vi "Vision Processing.vi"(4 "error in (no error)":errorcluster, 7 "Image Size":T4=enum."320x240") -> ()   [LabVIEW 2014]
doc: "This VI runs in parallel to other tasks. It gets images from the camera, processes them for color or shape and use that information to affect robot behavior."
uses:
  <vilib>/Rock Robotics/WPI/Camera/WPI_CameraImageSize.ctl
  <vilib>/Rock Robotics/WPI/Camera/WPI_CameraSettings Read MJPG.ctl
  Global Variables.vi
  Robot Global Data.vi
  <vilib>/Rock Robotics/WPI/Camera/WPI_CameraWhite Balance Values.ctl
  <vilib>/Rock Robotics/WPI/Camera/WPI_CameraExposure Values.ctl
  <vilib>/Rock Robotics/WPI/Camera/WPI_CameraFrameRate.ctl
  <vilib>/vision/NI_Vision_Development_Module.lvlib
  <vilib>/vision/Image Controls.llb/IMAQ Image.ctl
panel:
  in  "Instructions:":string="Use the tab immediately below to choose the image source. Update the camera settings or the image directory so that you have images or video to test with.\n\nCalibration:\nYou can update Color Component ranges directly, or by clicking and drawing a line across the upper third of a ball within the image -- example shown below-right.\n\nUse Debugging tab to view intermediate results. Adjust Std Dev multipliers and line to achieve the desired HSV upper and lower threshold limits.\n\nArea Size LImit is used to ignore objects too small or balls too far away to care about.\n\nTargets identifies how many of the top scores to return.\n\nThe Details tab contains center, radius, and score details of each object."
  in  "Tabbed Info":enum32{"Debugging", "Details"}(tab)
  in  "Annotations":enum16{"None", "Good", "All"}(ring)=enum."Good"
  out "Initial Mask":T1(plugin-control)
  out "Fitted Mask":T1(plugin-control)
  out "Ranked Objects":T2(array[cluster]) {"Score" format="%#.1g"}
  out "Image":T1(plugin-control)
  in  "Image Source":enum32{"Files", "Camera"}(tab)
  in  "List of image files":i32(listbox)
  in  "Image Directory":path=path "2014 Vision Target"
  in  "Camera Settings":T3={"fps"=15, "compression"=5, "Image Size"=enum."320x240"}
  in  "Camera IP":string="10.04.19.11"
  in  "Camera Address":string="192.168.0.90"
  out "Error":bool
  in  "Area Size Limit %":dbl=0.4 format="%#_13g"
  in  "Score Cutoff":dbl(slide)=70.58823529411765 scale=0.0..100.0
  out "loop time ms":u32
  in  "Targets":i32=3
  in  "Color Components":T5={"Hue"={45.217481128107224, 100.83905198430494}, "Sat"={154.78571428571428, 255.0}, "Val"={197.32142857142856, 255.0}} {"Val" scale=0.0..255.0; "Sat" scale=0.0..255.0; "Hue" scale=0.0..255.0 scale format="%#_3g"}
  in  "Std Devs":cluster{"Hue":dbl, "Sat":dbl, "Val":dbl}={"Hue"=4.0, "Sat"=6.0, "Val"=4.0}
  in  "Image Size 2":T4=enum."320x240"
  out "Blue 3":cluster{"Lower value":i32, "Upper value":i32}={"Lower value"=0, "Upper value"=255}
  out "Red":cluster{"Lower value":i32, "Upper value":i32}={"Lower value"=0, "Upper value"=255}
  out "Green 3":cluster{"Lower value":i32, "Upper value":i32}={"Lower value"=0, "Upper value"=255}
  in  "Threshold Distance":cluster{"Lower value":i32, "Upper value":i32}={"Lower value"=0, "Upper value"=255} {"Upper value" scale=0.0..255.0; "Lower value" scale=0.0..255.0}
  in  "Red Control":cluster{"Lower value":i32, "Upper value":i32}={"Lower value"=0, "Upper value"=255} {"Upper value" scale=0.0..255.0; "Lower value" scale=0.0..255.0}
  in  "Green Control":cluster{"Lower value":i32, "Upper value":i32}={"Lower value"=0, "Upper value"=255} {"Upper value" scale=0.0..255.0; "Lower value" scale=0.0..255.0}
  in  "Blue Control":cluster{"Lower value":i32, "Upper value":i32}={"Lower value"=0, "Upper value"=255} {"Upper value" scale=0.0..255.0; "Lower value" scale=0.0..255.0}
  in  "Images":T6(tab)=enum."5. Morphological Reconstruction"
  out "Source Image":T1(plugin-control)
  out "Threshold Image":T1(plugin-control)
  out "Distance Image":T1(plugin-control)
  out "Threshold Distance 2":T1(plugin-control)
  out "Reconstructed Image":T1(plugin-control)
  out "Red 2":cluster{"Lower value":i32, "Upper value":i32}={"Lower value"=0, "Upper value"=255}
  out "Blue 2":cluster{"Lower value":i32, "Upper value":i32}={"Lower value"=0, "Upper value"=255}
  out "Green 2":cluster{"Lower value":i32, "Upper value":i32}={"Lower value"=0, "Upper value"=255}
  in  "Blue":cluster{"Lower value":i32, "Upper value":i32}={"Lower value"=0, "Upper value"=255} {"Upper value" scale=0.0..255.0; "Lower value" scale=0.0..255.0}
  in  "Green":cluster{"Lower value":i32, "Upper value":i32}={"Lower value"=0, "Upper value"=255} {"Upper value" scale=0.0..255.0; "Lower value" scale=0.0..255.0}
  in  "Red or Hue Range":cluster{"Lower value":i32, "Upper value":i32}={"Lower value"=0, "Upper value"=255} {"Upper value" scale=0.0..255.0; "Lower value" scale=0.0..255.0}
  in  "Replace Value":sgl=1.0 format="%.2f"
  out "Image Dst Out":T1(plugin-control)
  out "Image Out":T1(plugin-control)
  # "Ranking Colors:\n1. green\n2. cyan\n3. magenta\n4. orange"
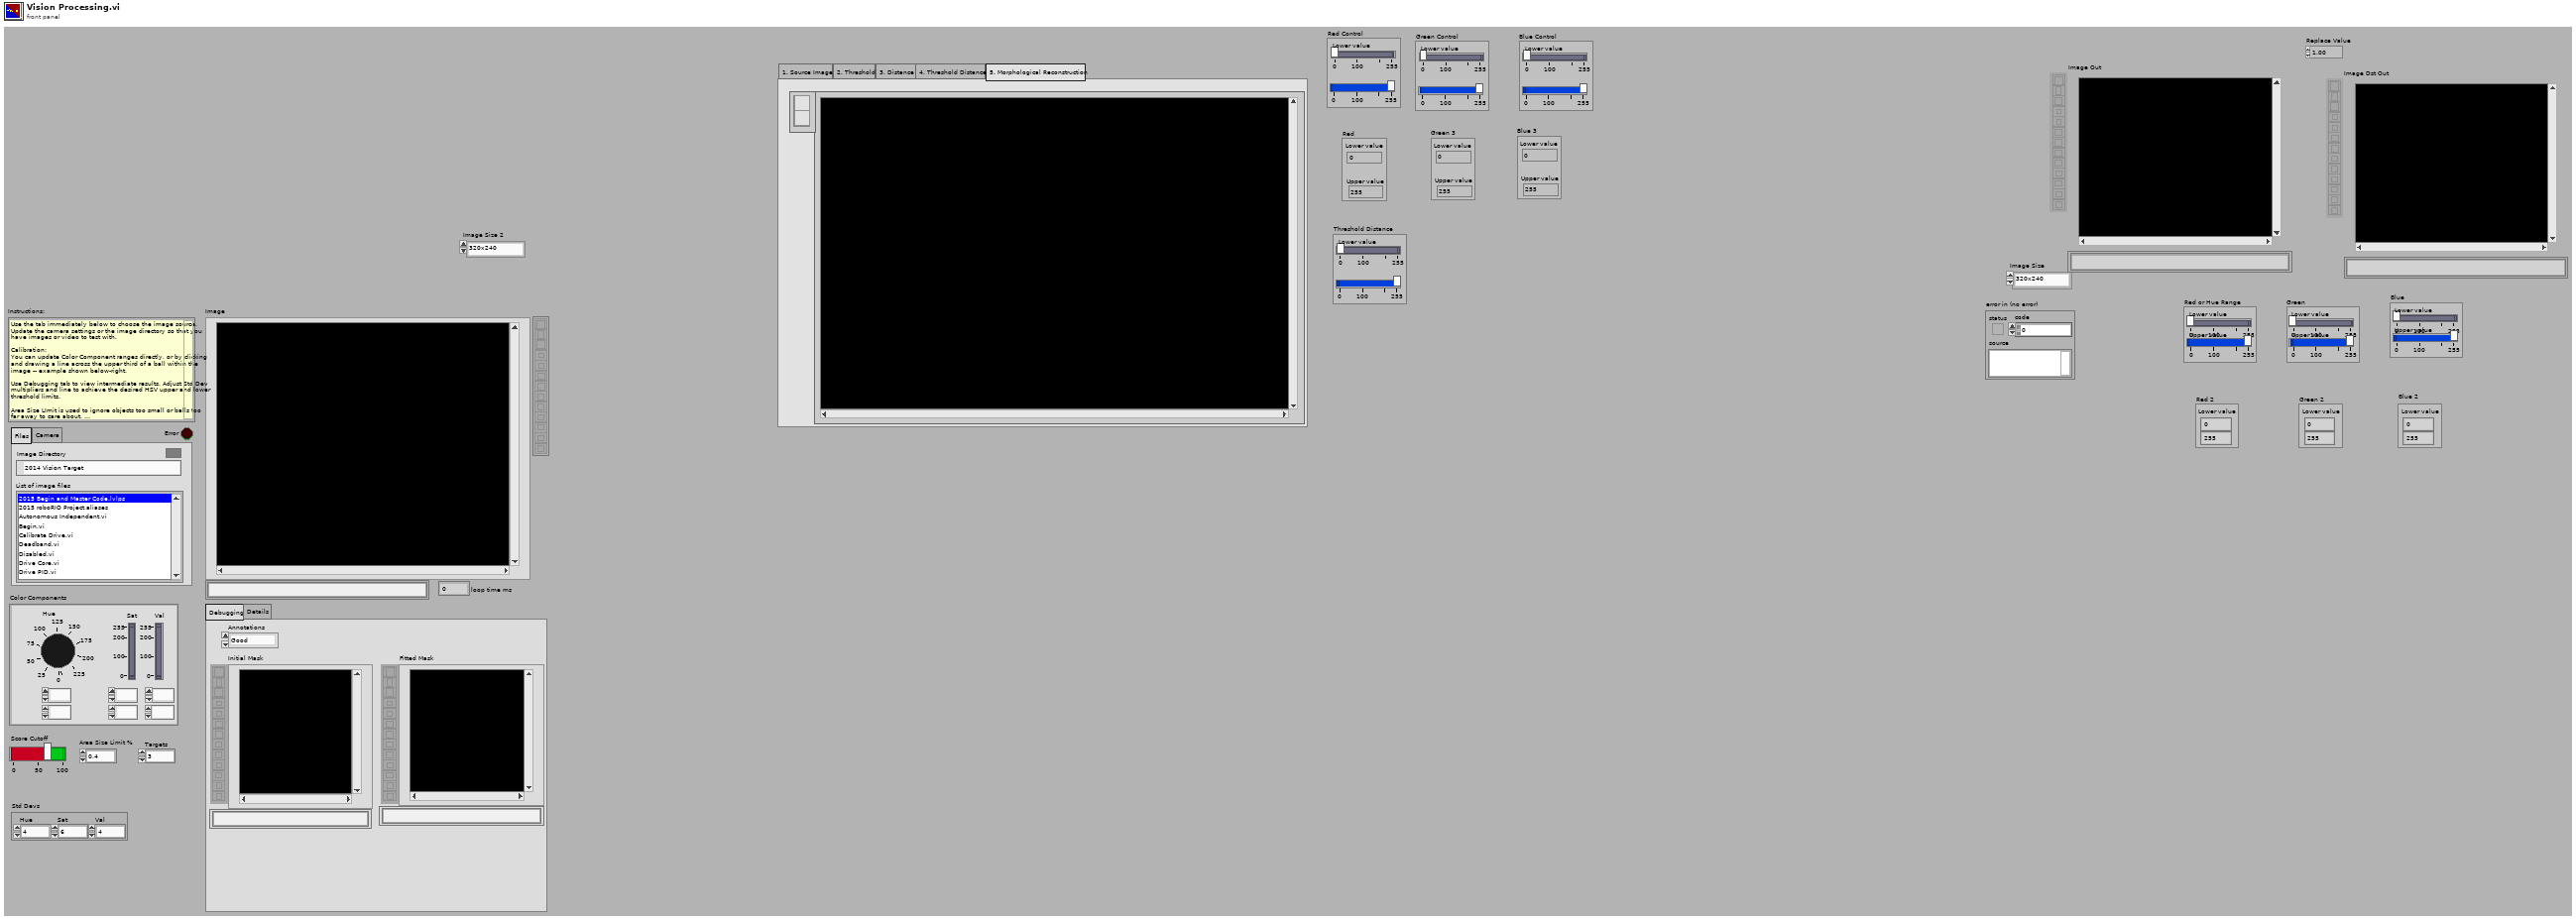
[diagram p1: front panel]
types:
  T1 = typedef "IMAQ Image.ctl" = refnum<image>
  T2 = cluster{"Score":sgl, "Fitted Circle":cluster{"Center":cluster{"X":sgl, "Y":sgl}, "Radius":dbl, "Circle Rect":cluster{"L":sgl, "T":sgl, "R":sgl, "B":sgl}, "Roundness":dbl, "SNR (dB)":dbl}, "Search Rect":cluster{"L":sgl, "T":sgl, "R":sgl, "B":sgl}, "Details":cluster{"Edge":sgl, "Area":sgl, "Circ":sgl, "Diam":sgl}}[]
  T3 = typedef "WPI_CameraSettings Read MJPG.ctl" = cluster{"fps":i32, "compression":i32, "Image Size":T4}
  T4 = typedef "WPI_CameraImageSize.ctl" = enum16{"640x480", "320x240", "160x120", "Custom"}
  T5 = cluster{"Hue":cluster{dbl, dbl}, "Sat":cluster{dbl, dbl}, "Val":cluster{dbl, dbl}}
  T6 = enum32{"1. Source Image", "2. Threshold", "3. Distance", "4. Threshold Distance", "5. Morphological Reconstruction"}
  T7 = typedef "WPI_CameraFrameRate.ctl" = u32
  T8 = typedef "WPI_CameraExposure Values.ctl" = enum16{"Auto", "Flicker-free 50 Hz", "Flicker-free 60 Hz", "Hold current", "Custom"}
  T9 = typedef "WPI_CameraWhite Balance Values.ctl" = enum16{"Auto", "Fixed indoor", "Fixed outdoor 1", "Fixed outdoor 2", "Fixed fluorescent 1", "Fixed fluorescent 2", "Hold current", "Custom"}
  T10 = typedef "WPI_CameraDevRef.ctl" = cluster{"Camera Address":string, "CameraStatus":errorcluster}
  T11 = typedef "Image Type" = u32
  T12 = cluster{"on/off":i32, "Fault 1":i32, "Fault 2":i32, "Fault 3":i32, "Fault 4":i32, "Inhibit 1":i32, "Inhibit 2":i32, "Inhibit 3":i32, "Inhibit 4":i32, "Limit 1":i32, "Limit 2":i32, "Limit 3":i32, "Limit 4":i32}
  T13 = cluster{"Fault 2":bool, "Fault 1":bool, "Fault 3":bool, "Fault 4":bool, "Fault 5":bool, "Fault 6":bool, "Fault 7":bool, "Fault 8":bool, "Fault 9":bool, "Fault 10":bool, "Fault 11":bool, "Fault 12":bool, "Fault 13":bool}
  T14 = cluster{"Circle Found":bool, "Fitted Circle":cluster{"Center":cluster{"X":sgl, "Y":sgl}, "Radius":dbl, "Center":cluster{"X":sgl, "Y":sgl}, "Radius":dbl, "Roundness":dbl, "Strength":dbl, "SNR (dB)":dbl}, "Array":dbl[], "Sorted Data":dbl[][]}[]
  T15 = cluster{cluster{dbl, dbl}, cluster{dbl, dbl}, cluster{dbl, dbl}}
  T16 = cluster{"Score":dbl, "Fitted Circle":cluster{"Center (Pixels)":cluster{"X":sgl, "Y":sgl}, "Radius (Pixels)":dbl, "Circle Rect":cluster{"Left":sgl, "Top":sgl, "Right":sgl, "Bottom":sgl}, "Roundness (RW)":dbl, "Average SNR (dB)":dbl}, "Search Rect":cluster{"Left":sgl, "Top":sgl, "Right":sgl, "Bottom":sgl}, "Details":cluster{"Edges":sgl, "Circ/Rect":sgl, "Diam/Diam":sgl, "Circularity":sgl}}[]
  T17 = cluster{"Score":dbl, "Fitted Circle":cluster{"Center (Pixels)":cluster{"X":sgl, "Y":sgl}, "Radius (Pixels)":dbl, "Circle Rect":cluster{"Left":sgl, "Top":sgl, "Right":sgl, "Bottom":sgl}, "Roundness (RW)":dbl, "Average SNR (dB)":dbl}, "Search Rect":cluster{"Left":sgl, "Top":sgl, "Right":sgl, "Bottom":sgl}, "Details":cluster{"Edges":sgl, "Circ/Rect":sgl, "Diam/Diam":sgl, "Circularity":sgl}}
  T18 = cluster{"Center (Pixels)":cluster{"X":sgl, "Y":sgl}, "Radius (Pixels)":dbl, "Circle Rect":cluster{"Left":sgl, "Top":sgl, "Right":sgl, "Bottom":sgl}, "Roundness (RW)":dbl, "Average SNR (dB)":dbl}
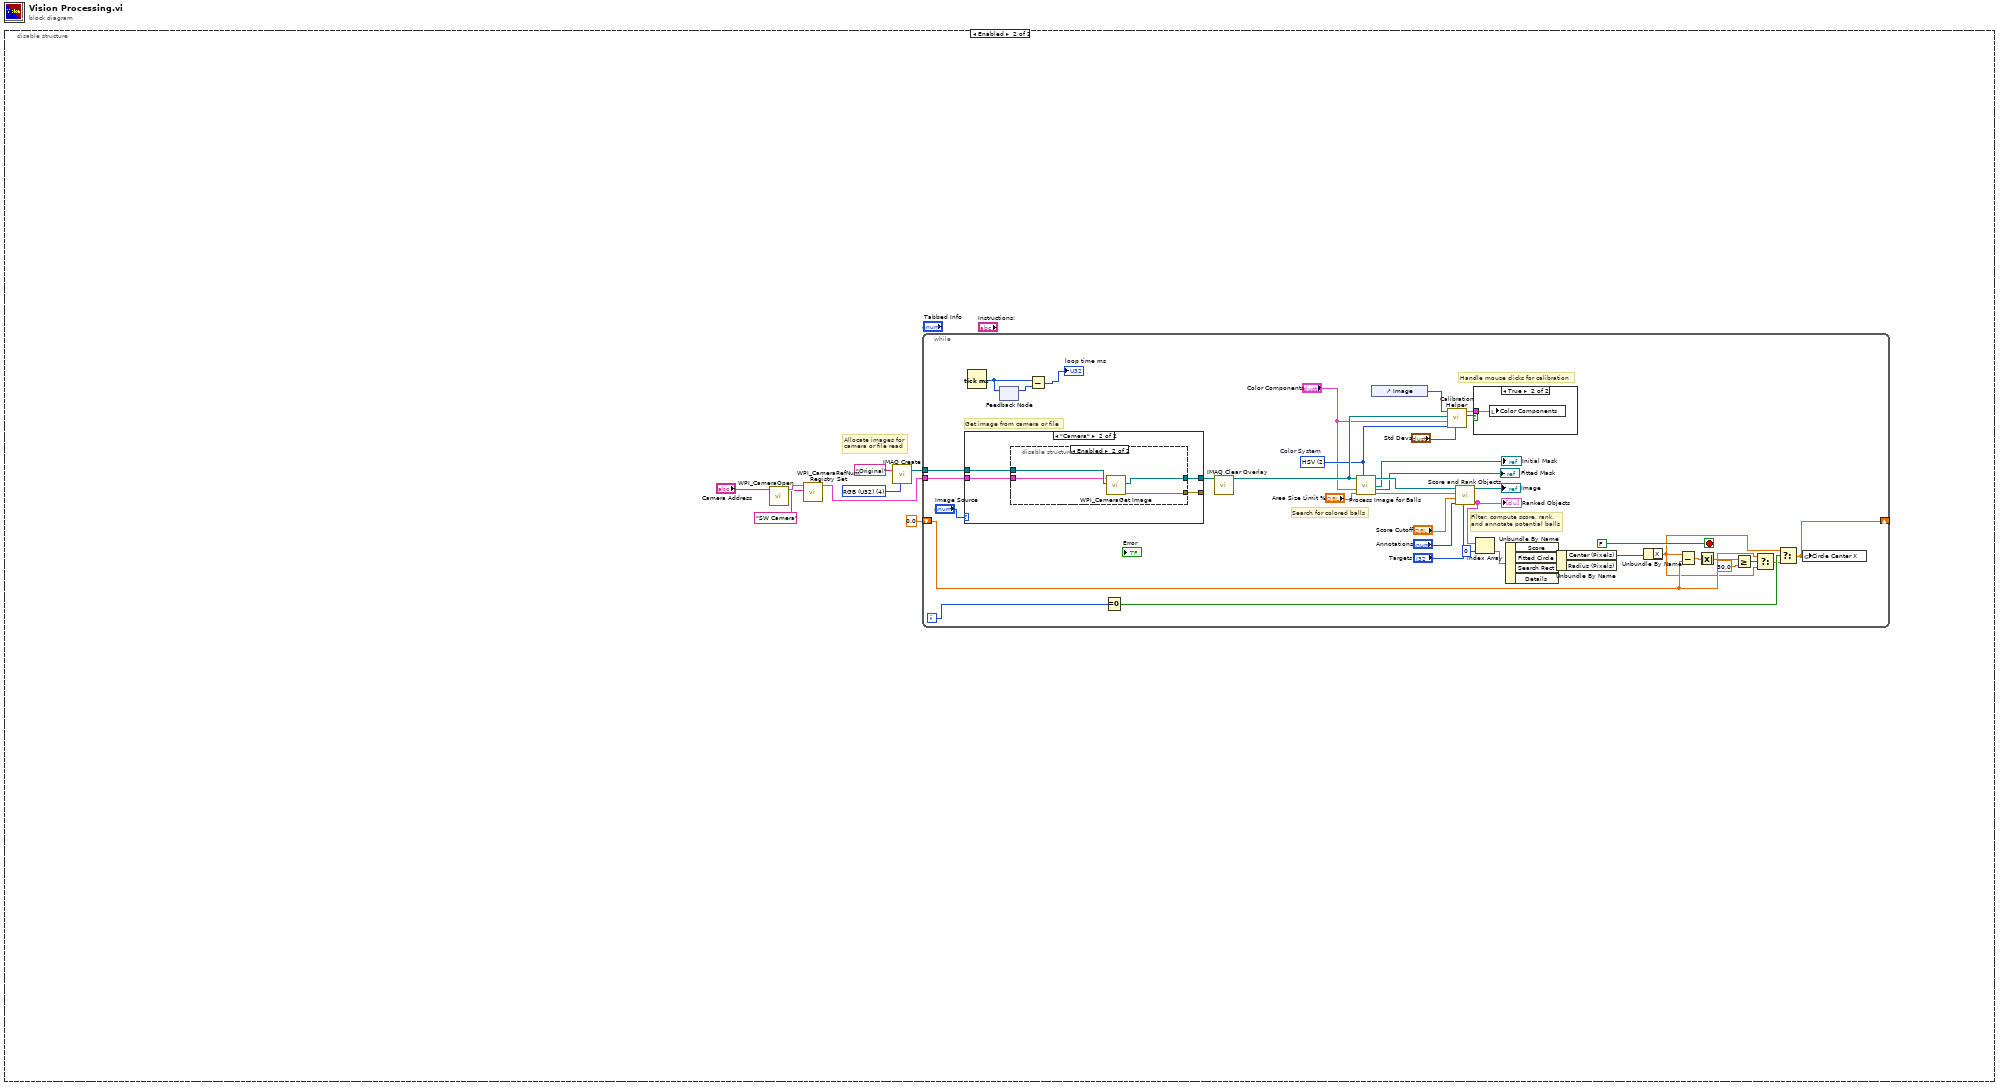
[diagram p0: block diagram]
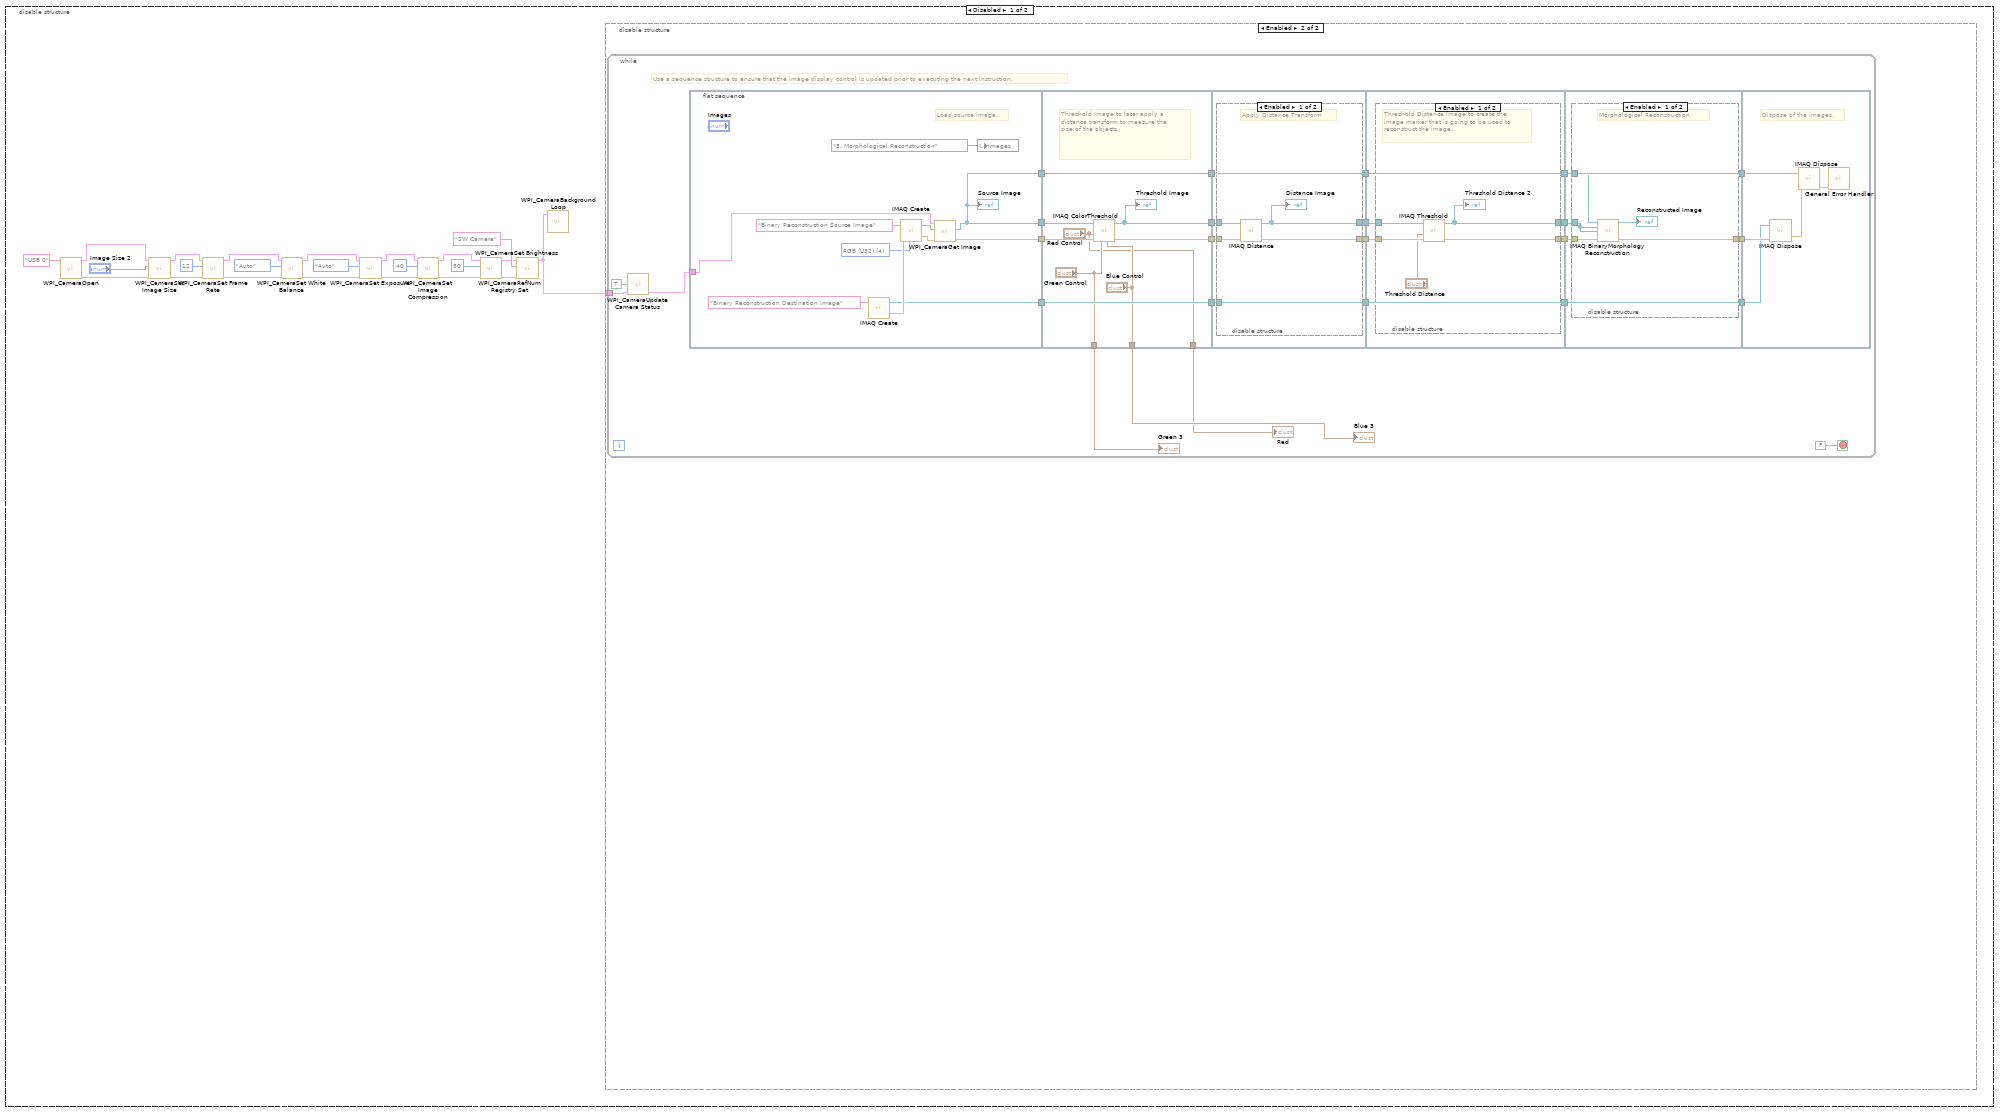
[diagram p2: hidden frame]
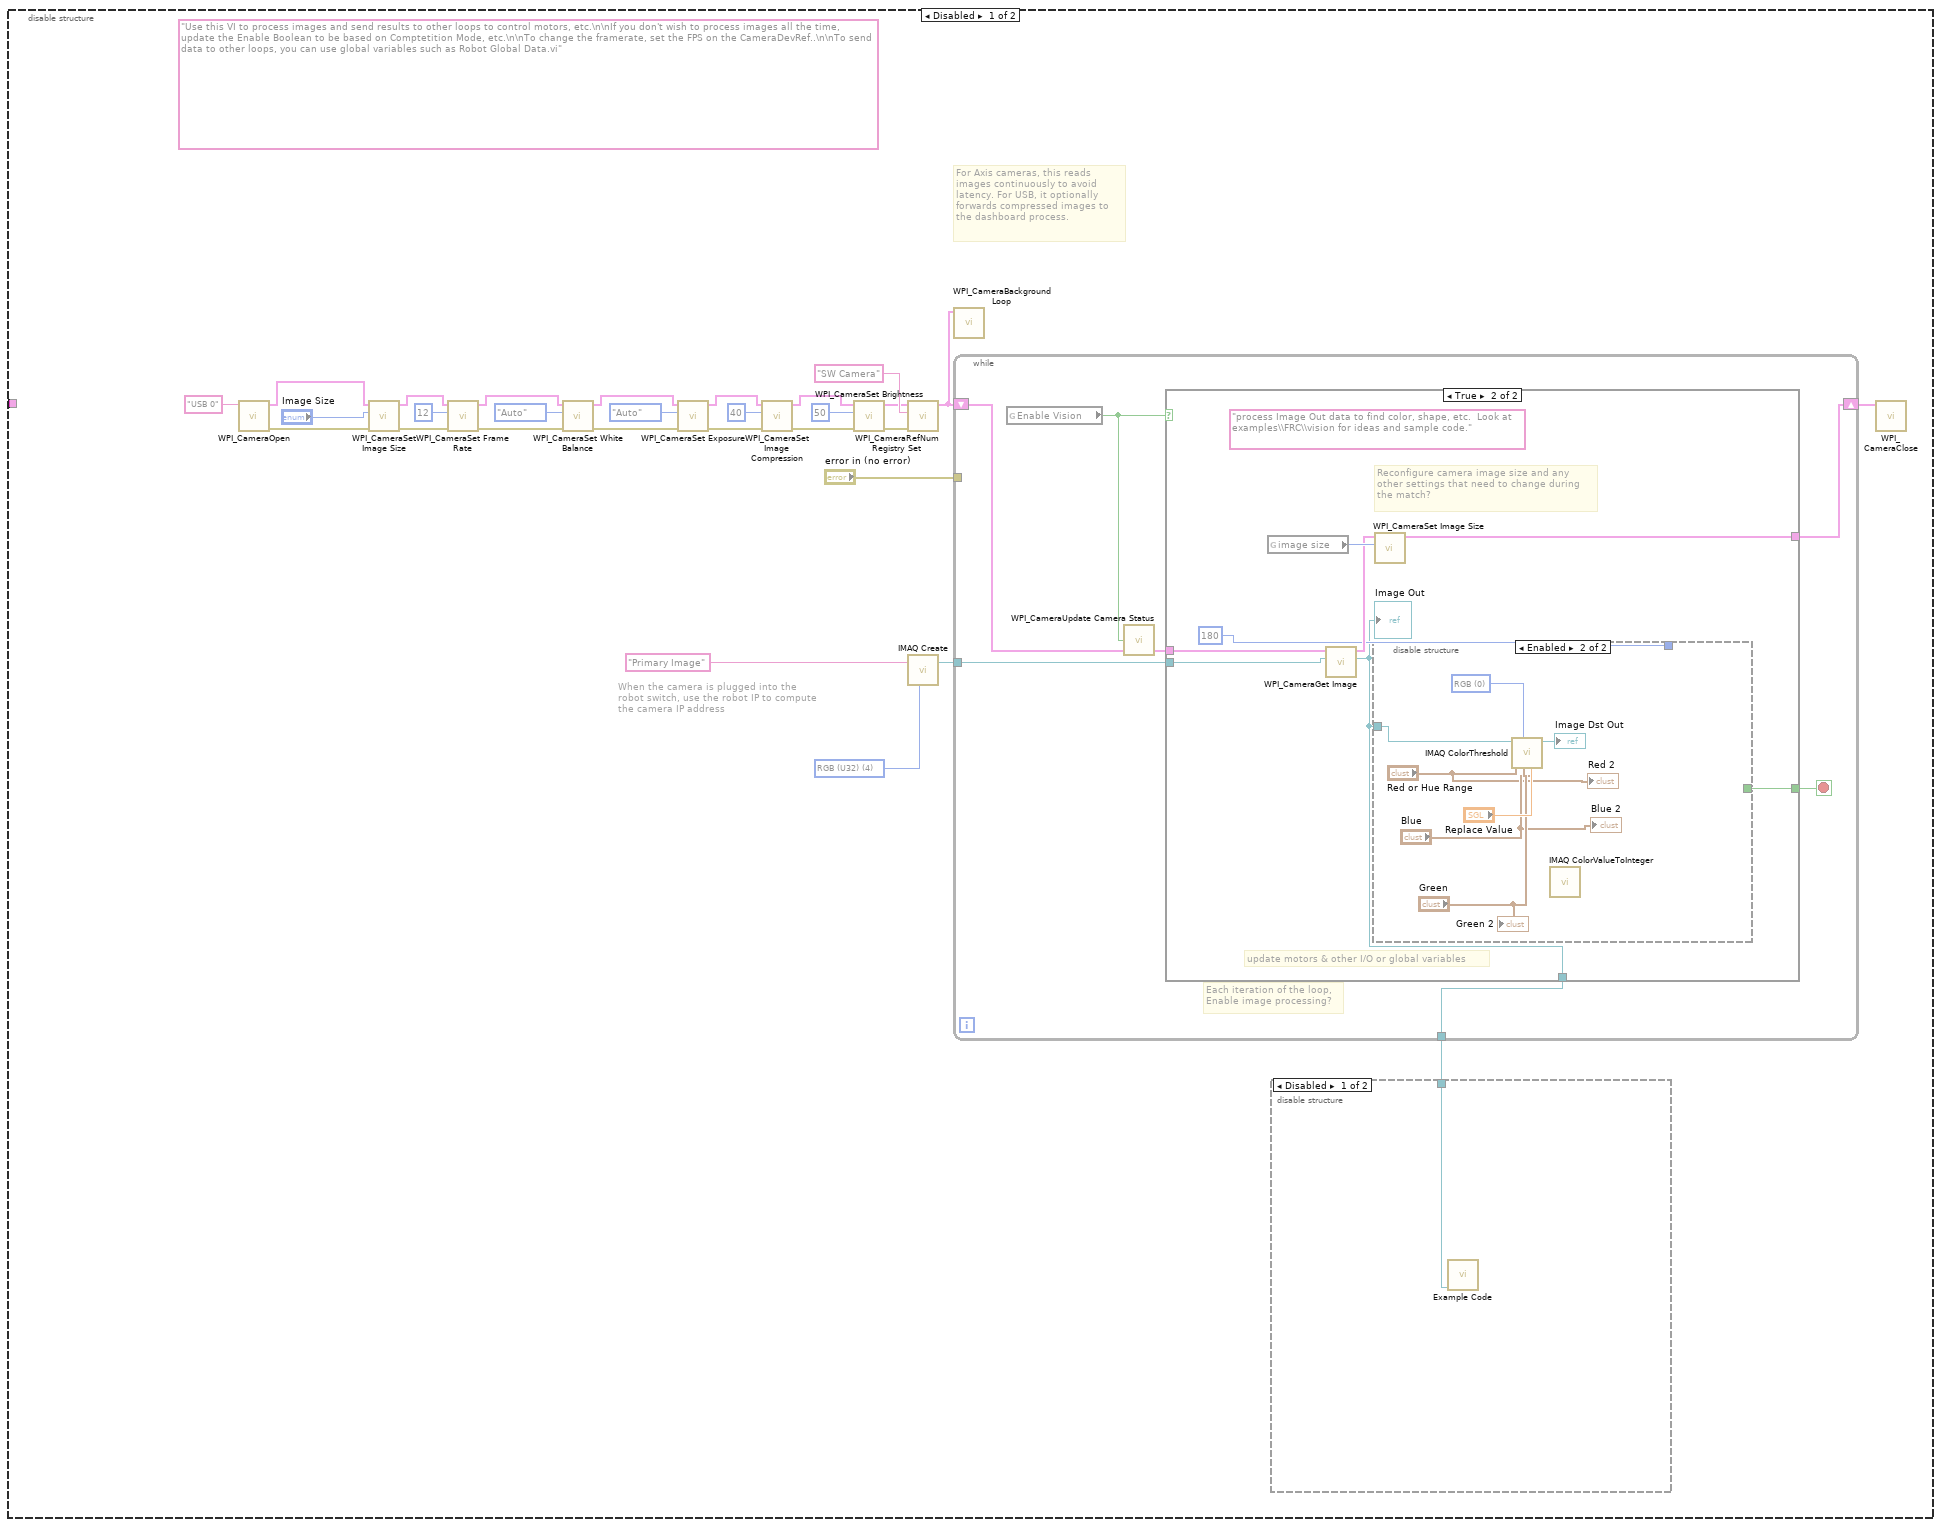
[diagram p3: hidden frame]
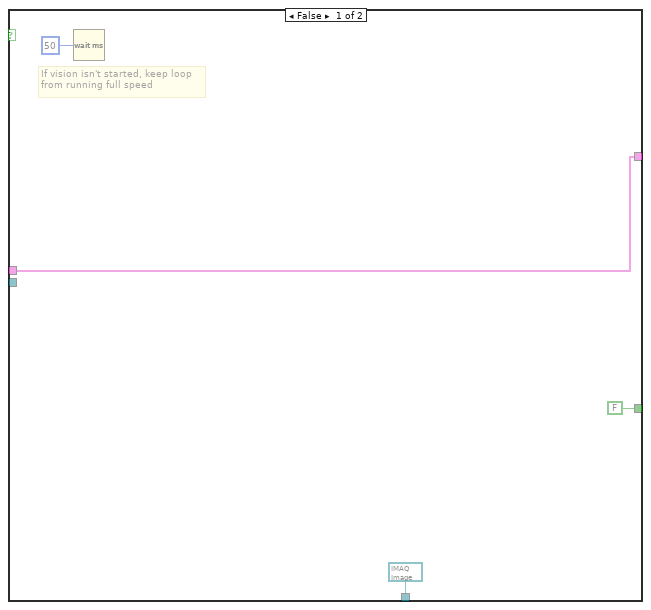
[diagram p5: hidden frame]
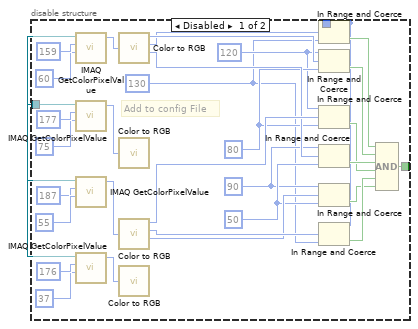
[diagram p6: hidden frame]
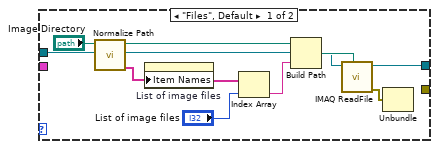
[diagram p11: hidden frame]
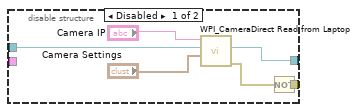
[diagram p12: hidden frame]
diagram:
  n1 = disable-structure shown="Enabled" {
    frame Disabled {
      n2 = call <vilib>:"WPI_CameraOpen.vi"("Camera Address"="USB 0" ("format string")) -> ("error out"=w14:errorcluster, "CameraDevRef"=w15:T10)  [unwired: 1 in, 8 out]
      n3 = call <vilib>:"WPI_CameraSet Image Size.vi"("error in (no error)"=w14, "Image Size"="Image Size 2", "CameraDevRef"=w15) -> ("error out"=w13:errorcluster, "CameraDevRef Out"=w16:T10)  [unwired: 1 in, 6 out]
      n4 = call <vilib>:"WPI_CameraSet Frame Rate.vi"("error in (no error)"=w13, "Frame Rate (fps)"=T7 12, "CameraDevRef"=w16) -> ("error out"=w12:errorcluster, "CameraDevRef Out"=w18:T10)  [unwired: 7 out]
      n5 = call <vilib>:"WPI_CameraSet White Balance.vi"("error in (no error)"=w12, "White Balance"=WPI_CameraWhite_Balance_Values."Auto", "CameraDevRef"=w18) -> ("error out"=w11:errorcluster, "CameraDevRef Out"=w17:T10)  [unwired: 1 in, 6 out]
      n6 = call <vilib>:"WPI_CameraSet Exposure.vi"("error in (no error)"=w11, "Exposure"=WPI_CameraExposure_Values."Auto", "CameraDevRef"=w17) -> ("error out"=w10:errorcluster, "CameraDevRef Out"=w20:T10)  [unwired: 1 in, 6 out]
      n7 = call <vilib>:"WPI_CameraSet Image Compression.vi"("error in (no error)"=w10, "Compression"=40, "CameraDevRef"=w20) -> ("error out"=w9:errorcluster, "CameraDevRef Out"=w19:T10)  [unwired: 7 out]
      n8 = call <vilib>:"WPI_CameraSet Brightness.vi"("error in (no error)"=w9, "Brightness"=50, "CameraDevRef"=w19) -> ("error out"=w7:errorcluster, "CameraDevRef Out"=w8:T10)  [unwired: 7 out]
      n9 = call <vilib>:"WPI_CameraRefNum Registry Set.vi"("error in (no error)"=w7, "refnum name"="SW Camera", "CameraDevRef"=w8) -> ("CameraDevRef"=w1:T10)  [unwired: 8 out]
      n10 = call <vilib>:"WPI_CameraBackground Loop.vi"("CameraDevRef"=w1) -> ()  [unwired: 11 in]
      n11 = disable-structure shown="Enabled" {
        disable-tunnel: w1 -> [_ w126]
        frame Disabled {
          (unwired) "Use this VI to process images and send results to other loops to control motors, etc.\n\nIf you don't wish to process images all the time, update the Enable Boolean to be based on Comptetition Mode, etc.\n\nTo change the framerate, set the FPS on the CameraDevRef..\n\nTo send data to other loops, you can use global variables such as Robot Global Data.vi"
          w52 = T11 4 items=["Grayscale (U8)", "Grayscale (I16)", "Grayscale (SGL)", "Complex (CSG)", "RGB (U32)", "HSL (U32)", "RGB (U64)"] ("Image Type")
          # "When the camera is plugged into the\nrobot switch, use the robot IP to compute\nthe camera IP address"
          # "For Axis cameras, this reads\nimages continuously to avoid\nlatency. For USB, it optionally\nforwards compressed images to\nthe dashboard process."
          n12 = call <vilib>:"WPI_CameraOpen.vi"("Camera Address"="USB 0" ("format string")) -> ("error out"=w40:errorcluster, "CameraDevRef"=w41:T10)  [unwired: 1 in, 8 out]
          n13 = call <vilib>:"WPI_CameraSet Image Size.vi"("error in (no error)"=w40, "Image Size"="Image Size", "CameraDevRef"=w41) -> ("error out"=w39:errorcluster, "CameraDevRef Out"=w42:T10)  [unwired: 1 in, 6 out]
          n14 = call <vilib>:"WPI_CameraSet Frame Rate.vi"("error in (no error)"=w39, "Frame Rate (fps)"=T7 12, "CameraDevRef"=w42) -> ("error out"=w38:errorcluster, "CameraDevRef Out"=w44:T10)  [unwired: 7 out]
          n15 = call <vilib>:"WPI_CameraSet White Balance.vi"("error in (no error)"=w38, "White Balance"=WPI_CameraWhite_Balance_Values."Auto", "CameraDevRef"=w44) -> ("error out"=w37:errorcluster, "CameraDevRef Out"=w43:T10)  [unwired: 1 in, 6 out]
          n16 = call <vilib>:"WPI_CameraSet Exposure.vi"("error in (no error)"=w37, "Exposure"=WPI_CameraExposure_Values."Auto", "CameraDevRef"=w43) -> ("error out"=w36:errorcluster, "CameraDevRef Out"=w46:T10)  [unwired: 1 in, 6 out]
          n17 = call <vilib>:"WPI_CameraSet Image Compression.vi"("error in (no error)"=w36, "Compression"=40, "CameraDevRef"=w46) -> ("error out"=w35:errorcluster, "CameraDevRef Out"=w45:T10)  [unwired: 7 out]
          n18 = call <vilib>:"WPI_CameraSet Brightness.vi"("error in (no error)"=w35, "Brightness"=50, "CameraDevRef"=w45) -> ("error out"=w33:errorcluster, "CameraDevRef Out"=w34:T10)  [unwired: 7 out]
          n19 = call <vilib>:"WPI_CameraRefNum Registry Set.vi"("error in (no error)"=w33, "refnum name"="SW Camera", "CameraDevRef"=w34) -> ("CameraDevRef"=w29:T10)  [unwired: 8 out]
          n20 = call "IMAQ Create"("Image Name"="Primary Image", "Image Type"=w52) -> ("New Image"=w50:T1)  [unwired: 2 in, 2 out]
          n21 = call <vilib>:"WPI_CameraBackground Loop.vi"("CameraDevRef"=w29) -> ()  [unwired: 11 in]
          n22 = while {
            shift-right: [w74] -> w27
            shift-left: w29 -> [w72]
            tunnel: w50 -> [w73]
            tunnel: "error in (no error)" -> [_]
            tunnel: [w68] -> w24
            stop <- w69 stop-if-true
            # "Each iteration of the loop,\nEnable image processing?"
            n23 = global read "Robot Global Data.vi" "Enable Vision"() -> (w70:bool)
            n24 = call <vilib>:"WPI_CameraUpdate Camera Status.vi"("CameraDevRef In"=w72, "Enable Vision"=w70) -> ("CameraDevRef Out"=w71:T10)  [unwired: 3 in]
            n25 = case shown="True" w70 {
              tunnel: w73 -> [_ w85]
              tunnel: [w78 w86] -> w74
              tunnel: w71 -> [w78 w83]
              tunnel: [FALSE w80] -> w69
              tunnel: [T1 refnum ("Image Out") w79] -> w68
              frame False {
                # "If vision isn't started, keep loop\nfrom running full speed"
                n26 = Wait (ms)(milliseconds to wait=u32 50) -> ()  [unwired: 1 out]
              }
              frame True {
                (unwired) "process Image Out data to find color, shape, etc.  Look at examples\\FRC\\vision for ideas and sample code."
                # "update motors & other I/O or global variables"
                # "Reconfigure camera image size and any\nother settings that need to change during\nthe match?"
                n27 = global read "Robot Global Data.vi" "image size"() -> (w84:T4)
                n28 = call <vilib>:"WPI_CameraGet Image.vi"("Image"=w85, "CameraDevRef"=w83) -> ("Image Out"=w79:T1, "CameraDevRef Out"=w82:T10)  [unwired: 1 in, 7 out]
                "Image Out" <- w79
                n29 = disable-structure shown="Enabled" {
                  disable-tunnel: u8 180 ("x") -> [w87 _]
                  disable-tunnel: [w89 _] -> w80
                  disable-tunnel: w79 -> [w88 w125]
                  frame Disabled {
                    w90 = u8 130 ("x")
                    w91 = u8 90 ("x")
                    w92 = u8 50 ("x")
                    w93 = u8 120 ("x")
                    w94 = u8 80 ("x")
                    # "Add to config File"
                    n30 = call "IMAQ GetColorPixelValue"("Y Coordinate"=60, "X Coordinate"=159, "Image"=w88) -> ("Pixel Value (U32)"=w108:u32)  [unwired: 1 in, 2 out]
                    n31 = call "IMAQ GetColorPixelValue"("Y Coordinate"=75, "X Coordinate"=177, "Image"=w88) -> ("Pixel Value (U32)"=w109:u32)  [unwired: 1 in, 2 out]
                    n32 = call "IMAQ GetColorPixelValue"("Y Coordinate"=55, "X Coordinate"=187, "Image"=w88) -> ("Pixel Value (U32)"=w110:u32)  [unwired: 1 in, 2 out]
                    n33 = call "IMAQ GetColorPixelValue"("Y Coordinate"=37, "X Coordinate"=176, "Image"=w88) -> ("Pixel Value (U32)"=w107:u32)  [unwired: 1 in, 2 out]
                    n34 = call <vilib>:"Color to RGB.vi"("Color"=w108) -> ("Resolved Color"=w106:u32, "R"=w104:u8, "G"=w103:u8)  [unwired: 1 out]
                    n35 = call <vilib>:"Color to RGB.vi"("Color"=w109) -> ()  [unwired: 4 out]
                    n36 = call <vilib>:"Color to RGB.vi"("Color"=w110) -> ("Resolved Color"=w105:u32, "R"=w102:u8, "G"=w101:u8)  [unwired: 1 out]
                    n37 = call <vilib>:"Color to RGB.vi"("Color"=w107) -> ()  [unwired: 4 out]
                    n38 = In Range and Coerce(upper limit=w87, x=w104, lower limit=w90) -> (In Range?=w100:bool)  [unwired: 1 out]
                    n39 = In Range and Coerce(upper limit=w93, x=w106, lower limit=w94) -> (In Range?=w99:bool)  [unwired: 1 out]
                    n40 = In Range and Coerce(upper limit=w93, x=w105, lower limit=w94) -> (In Range?=w97:bool)  [unwired: 1 out]
                    n41 = In Range and Coerce(upper limit=w91, x=w103, lower limit=w92) -> (In Range?=w98:bool)  [unwired: 1 out]
                    n42 = In Range and Coerce(upper limit=w91, x=w101, lower limit=w92) -> (In Range?=w95:bool)  [unwired: 1 out]
                    n43 = In Range and Coerce(upper limit=w87, x=w102, lower limit=w90) -> (In Range?=w96:bool)  [unwired: 1 out]
                    n44 = Compound Arithmetic op=AND(w100, w99, w98, w97, w96, w95) -> (w89:bool)
                  }
                  frame Enabled {
                    w122 = u16 0 items=["RGB", "HSL", "HSV", "HSI"] ("Color Mode")
                    n45 = call "IMAQ ColorThreshold"("Blue or Luma or Val or Inten Range"="Blue", "Replace Value"="Replace Value", "Green or Sat Range"="Green", "Color Mode"=w122, "Red or Hue Range"="Red or Hue Range", "Image Src"=w125) -> ("Image Dst Out"=→"Image Dst Out":T1)  [unwired: 4 in, 1 out]
                    n46 = call "IMAQ ColorValueToInteger"() -> ()  [unwired: 5 in, 4 out]
                    "Green 2" <- "Green"
                    "Blue 2" <- "Blue"
                    "Red 2" <- "Red or Hue Range"
                  }
                }
                n47 = call <vilib>:"WPI_CameraSet Image Size.vi"("Image Size"=w84, "CameraDevRef"=w82) -> ("CameraDevRef Out"=w86:T10)  [unwired: 2 in, 7 out]
              }
            }
          }
          n48 = disable-structure shown="Disabled" {
            disable-tunnel: w24 -> [w53 _]
            frame Disabled {
              n49 = call "Example Code.vi"("Image"=w53) -> ("Red Color Array"=w66:u32[][], "Black Color Array"=w67:u32[][], "Green Color Spectrum"=w61:dbl[][], "Orange Color Spectrum"=w60:dbl[][], "Refnum out"=w56:T1, "Orange Color Array"=w65:u32[][], "Red Color Spectrum"=w59:dbl[][], "Green Color Array"=w64:u32[][], "Black Color Spectrum"=w58:dbl[][], "Stop"=w63:bool, "Expected Pattern"=w57:T12, "Delay (s.)"=w62:dbl, "Global Status"=w54:bool, "Pass/Fail"=w55:T13)  [unwired: 1 in]
            }
            frame Enabled {
            }
          }
          n50 = call <vilib>:"WPI_CameraClose.vi"("CameraDevRef"=w27) -> ()  [unwired: 1 in, 10 out]
        }
        frame Enabled {
          n51 = while {
            tunnel: w126 -> [w128]
            stop <- FALSE stop-if-true
            # "Use a sequence structure to ensure that the image display control is updated prior to executing the next instruction."
            n52 = call <vilib>:"WPI_CameraUpdate Camera Status.vi"("CameraDevRef In"=w128, "Enable Vision"=TRUE) -> ("CameraDevRef Out"=w127:T10)  [unwired: 3 in]
            n53 = flat-sequence {
              tunnel: [w155] -> w152
              tunnel: [w156] -> w151
              tunnel: [w160] -> w150
              tunnel: [w156] -> w149
              tunnel: w127 -> [w153]
              tunnel: w152 -> [w171]
              tunnel: w151 -> [w172]
              tunnel: w150 -> [w168]
              tunnel: [w170] -> w148
              tunnel: [w169] -> w147
              tunnel: [w168] -> w146
              tunnel: [w167] -> w145
              tunnel: w149 -> [w167]
              tunnel: ["Green Control"] -> w133
              tunnel: ["Blue Control"] -> w132
              tunnel: ["Red Control"] -> w131
              tunnel: w148 -> [w177]
              tunnel: w147 -> [w178]
              tunnel: [w176] -> w144
              tunnel: [w175] -> w143
              tunnel: w146 -> [w173]
              tunnel: [w174] -> w142
              tunnel: w145 -> [w174]
              tunnel: [w173] -> w141
              tunnel: w144 -> [w188]
              tunnel: w143 -> [w187]
              tunnel: [w186] -> w140
              tunnel: [w185] -> w139
              tunnel: w142 -> [w185]
              tunnel: [w184] -> w138
              tunnel: [w183] -> w137
              tunnel: w141 -> [w183]
              tunnel: w140 -> [w198]
              tunnel: w139 -> [w195]
              tunnel: w138 -> [w197]
              tunnel: [w196] -> w136
              tunnel: [w195] -> w135
              tunnel: [w194] -> w134
              tunnel: w137 -> [w194]
              tunnel: w136 -> [w208]
              tunnel: w135 -> [w207]
              tunnel: w134 -> [w204]
              frame #0 {
                w158 = T11 4 items=["Grayscale (U8)", "Grayscale (I16)", "Grayscale (SGL)", "Complex (CSG)", "RGB (U32)", "HSL (U32)", "RGB (U64)", "Grayscale (U16)"] ("Image Type")
                # "Load source image."
                n54 = call "IMAQ Create"("Image Name"="Binary Reconstruction Destination Image") -> ("New Image"=w160:T1, "error out"=w161:errorcluster)  [unwired: 3 in, 1 out]
                n55 = call "IMAQ Create"("Image Name"="Binary Reconstruction Source Image", "Image Type"=w158, "error in (no error)"=w161) -> ("New Image"=w157:T1, "error out"=w154:errorcluster)  [unwired: 1 in, 1 out]
                n56 = call <vilib>:"WPI_CameraGet Image.vi"("error in (no error)"=w154, "Image"=w157, "CameraDevRef"=w153) -> ("error out"=w155:errorcluster, "Image Out"=w156:T1)  [unwired: 7 out]
                "Source Image" <- w156
                n57 = local write "Images"(T6."5. Morphological Reconstruction" ("Images")) -> ()
              }
              frame #1 {
                # "Threshold Image to later apply a distance transform to measure the size of the objects."
                n58 = call "IMAQ ColorThreshold"("Blue or Luma or Val or Inten Range"="Blue Control", "Green or Sat Range"="Green Control", "error in (no error)"=w171, "Red or Hue Range"="Red Control", "Image Src"=w172) -> ("error out"=w170:errorcluster, "Image Dst Out"=w169:T1)  [unwired: 5 in]
                "Threshold Image" <- w169
              }
              frame #2 {
                n59 = disable-structure shown="Enabled" {
                  disable-tunnel: w178 -> [w182 _]
                  disable-tunnel: w177 -> [w181 _]
                  disable-tunnel: [w180 _] -> w176
                  disable-tunnel: [w179 _] -> w175
                  disable-tunnel: w173 -> [_ _]
                  frame Enabled {
                    # "Apply Distance Transform"
                    n60 = call "IMAQ Distance"("error in (no error)"=w181, "Image Src"=w182) -> ("error out"=w179:errorcluster, "Image Dst Out"=w180:T1)  [unwired: 2 in, 2 out]
                    "Distance Image" <- w180
                  }
                  frame Disabled {
                  }
                }
              }
              frame #3 {
                n61 = disable-structure shown="Enabled" {
                  disable-tunnel: w188 -> [w193 _]
                  disable-tunnel: w187 -> [w192 _]
                  disable-tunnel: [w191 _] -> w186
                  disable-tunnel: [w190 _] -> w184
                  frame Enabled {
                    # "Threshold Distance Image to create the image marker that is going to be used to reconstruct the image."
                    n62 = call "IMAQ Threshold"("error in (no error)"=w192, "Range"="Threshold Distance", "Image Src"=w193) -> ("error out"=w190:errorcluster, "Image Dst Out"=w191:T1)  [unwired: 3 in, 4 out]
                    "Threshold Distance 2" <- w191
                  }
                  frame Disabled {
                  }
                }
              }
              frame #4 {
                n63 = disable-structure shown="Enabled" {
                  disable-tunnel: w198 -> [w203 _]
                  disable-tunnel: w197 -> [w201 _]
                  disable-tunnel: [w200 _] -> w196
                  disable-tunnel: w195 -> [w199 _]
                  frame Enabled {
                    # "Morphological Reconstruction"
                    n64 = call "IMAQ BinaryMorphology Reconstruction"("Image Src"=w199, "Image Dst"=w203, "Image Marker"=w203, "error in (no error)"=w201) -> ("Image Dst Out"=→"Reconstructed Image":T1, "error out"=w200:errorcluster)  [unwired: 4 in, 6 out]
                  }
                  frame Disabled {
                  }
                }
              }
              frame #5 {
                # "Dispose of the images."
                n65 = call "IMAQ Dispose"("Image"=w204, "error in (no error)"=w208) -> ("error out"=w206:errorcluster)  [unwired: 1 in, 3 out]
                n66 = call "IMAQ Dispose"("Image"=w207, "error in (no error)"=w206) -> ("error out"=w205:errorcluster)  [unwired: 1 in, 3 out]
                n67 = call <vilib>:"General Error Handler.vi"("error in (no error)"=w205) -> ()  [unwired: 10 in, 5 out]
              }
            }
            "Green 3" <- w133
            "Red" <- w131
            "Blue 3" <- w132
          }
        }
      }
    }
    frame Enabled {
      w216 = T11 4 items=["Grayscale (U8)", "Grayscale (I16)", "Grayscale (SGL)", "Complex (CSG)", "RGB (U32)", "HSL (U32)", "RGB (U64)", "Grayscale (U16)"] ("Image Type")
      # "Allocate images for\ncamera or file read"
      n68 = call <vilib>:"WPI_CameraOpen.vi"("Camera Address"="Camera Address") -> ("CameraDevRef"=w213:T10)  [unwired: 9 in, 1 out]
      n69 = call <vilib>:"WPI_CameraRefNum Registry Set.vi"("refnum name"="SW Camera", "CameraDevRef"=w213) -> ("CameraDevRef"=w211:T10)  [unwired: 8 in, 1 out]
      n70 = call "IMAQ Create"("Image Name"="Original", "Image Type"=w216) -> ("New Image"=w214:T1)  [unwired: 3 in, 1 out]
      n71 = while {
        tunnel: w214 -> [w252]
        tunnel: w211 -> [w233]
        shift-right: [w217] -> _
        shift-left: sgl 0.0 ("X") -> [w222]
        i -> [w221]
        stop <- FALSE stop-if-true
        w239 = u16 2 items=["RGB", "HSL", "HSV", "HSI"]  # Color System
        # "Handle mouse clicks for calibration"
        # "Search for colored balls"
        # "Filter, compute score, rank,\nand annotate potential balls"
        # "Get image from camera or file"
        n72 = case shown="\"Camera\"" "Image Source" {
          tunnel: [w262 w267] -> w255
          tunnel: w252 -> [w261 w268]
          tunnel: [_ w269] -> _
          tunnel: w233 -> [_ w266]
          frame "Files", Default {
            n73 = call "Normalize Path.vi"("Image Directory"="Image Directory") -> ("Filenames"=w259:string[], "Path"=w257:path)  [unwired: 9 in]
            n74 = property on="List of image files" class="LstBox (strict)"("Item Names"=w259) -> ()  [unwired: 2 in, 2 out]
            n75 = Index Array(array=w259, index="List of image files") -> (element=w264:string)
            n76 = Build Path(base path=w257, name or relative path=w264) -> (appended path=w263:path)
            n77 = call "IMAQ ReadFile"("File Path"=w263, "Image"=w261) -> ("error out"=w260:errorcluster, "Image Out"=w262:T1)  [unwired: 5 in, 3 out]
            n78 = Unbundle(w260) -> ()  [unwired: 3 out]
          }
          frame "Camera" {
            n79 = disable-structure shown="Enabled" {
              disable-tunnel: [w275 w277] -> w269
              disable-tunnel: w268 -> [w273 w279]
              disable-tunnel: [w271 w278] -> w267
              disable-tunnel: w266 -> [_ w276]
              frame Disabled {
                n80 = call <vilib>:"WPI_CameraDirect Read from Laptop.vi"("Camera Settings"="Camera Settings", "Image"=w273, "address"="Camera IP") -> ("error out"=w270:errorcluster, "Image Out"=w271:T1)  [unwired: 7 in]
                n81 = Not(x=w270) -> (.not. x?=w275:bool)
              }
              frame Enabled {
                n82 = call <vilib>:"WPI_CameraGet Image.vi"("Image"=w279, "CameraDevRef"=w276) -> ("error out"=w277:errorcluster, "Image Out"=w278:T1)  [unwired: 1 in, 7 out]
              }
            }
          }
        }
        n83 = Tick Count (ms)() -> (millisecond timer value=w251:u32)
        n84 = feedback #1() -> (w250:u32)  [unwired: 1 in]
        n85 = feedback-in #1(w251) -> ()
        n86 = Subtract(x=w251, y=w250) -> (x-y=→"loop time ms":u32)
        n87 = Equal To 0?(x=w221) -> (x = 0?=w220:bool)
        n88 = call "IMAQ Clear Overlay"("Image"=w255) -> ("Image Out"=w246:T1)  [unwired: 9 in, 1 out]
        n89 = call "Process Image for Balls.vi"("Src Image"=w246, "Color Mode 2"=w239, "Color"="Color Components", "Area Cutoff %"="Area Size Limit %") -> ("Src Image Out"=w244:T1, "First Threshold"=→"Initial Mask":T1, "Fitted"=→"Fitted Mask":T1, "Potential"=w243:T14)  [unwired: 8 in]
        n90 = control-ref of="Image"() -> (w238:refnum<vi>)
        n91 = call "Calibration Helper.vi"("Std Devs"="Std Devs", "Color Mode"=w239, "Color Components"="Color Components", "Image"=w246, "Image Ctl Refnum"=w238) -> ("Changed"=w235:bool, "output color"=w237:T15)  [unwired: 5 in]
        n92 = call "Score and Rank Objects.vi"("Targets"="Targets", "Annotations"="Annotations", "Score Limit"="Score Cutoff", "Object Info"=w243, "Image in"=w244) -> ("Object Info"=w231:T16, "Annotated Image"=→"Image":T1)  [unwired: 5 in]
        "Ranked Objects" <- w231
        n93 = case shown="True" w235 {
          tunnel: w237 -> [_ w256]
          frame False {
          }
          frame True {
            n94 = local write "Color Components"(w256) -> ()
          }
        }
        n95 = Index Array(array=w231, index=0) -> (element=w229:T17)
        n96 = Unbundle By Name(w229) -> ("Fitted Circle"=w228:T18)  [unwired: 3 out]
        n97 = Unbundle By Name(w228) -> ("Center (Pixels)"=w227:cluster{"X":sgl, "Y":sgl})  [unwired: 1 out]
        n98 = Unbundle By Name(w227) -> ("X"=w219:sgl)
        n99 = Subtract(x=w219, y=w222) -> (x-y=w226:sgl)
        n100 = Absolute Value(x=w226) -> (abs(x)=w225:sgl)
        n101 = Greater Or Equal?(x=w225, y=sgl 30.0) -> (x >= y?=w223:bool)
        n102 = Select(t=w222, s=w223, f=w219) -> (s? t:f=w218:sgl)
        n103 = Select(t=w219, s=w220, f=w218) -> (s? t:f=w217:sgl)
        n104 = global write "Global Variables.vi" "Circle Center X"(w217) -> ()
      }
    }
  }
